vi "Set H Mode Torque.vi"(8 "error in (no error)":errorcluster, 10 "Torque_Reference_H":dbl, 11 "TCP modebus instance in":refnum<class "Modbus Master.lvclass">[](array[class])) -> (0 "error out":errorcluster, 3 "TCP modebus instance out":refnum<class "Modbus Master.lvclass">[](array[class]))   [LabVIEW 2025]
uses:
  <vilib>/Modbus/master/Modbus Master.lvclass
  C:/Program Files/National Instruments/LabVIEW 2025/vi.lib/Modbus/subvis/Modbus API/Modbus API.lvclass
  <vilib>/Modbus/subvis/Modbus API/Modbus API.lvclass/Modbus API.ctl
  <vilib>/Modbus/subvis/Transmission Data Unit (ADU)/Transmission Data Unit/Transmission Data Unit.lvclass/Transmission Data Unit.ctl
  <vilib>/Modbus/master/Data Access/Unit ID/Set Unit ID Property.vi
  <vilib>/Modbus/subvis/Transmission Data Unit (ADU)/Transmission Data Unit/Data Access/Unit ID/Write Unit ID.vi
  <vilib>/Modbus/subvis/Modbus API/Read Transmission Data Unit.vi
  <vilib>/Modbus/subvis/Modbus API/Write Transmission Data Unit.vi
  <vilib>/Modbus/subvis/Transmission Data Unit (ADU)/Transmission Data Unit/Transmission Data Unit.lvclass
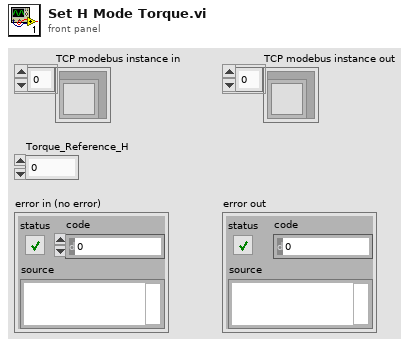
[diagram p1: front panel]
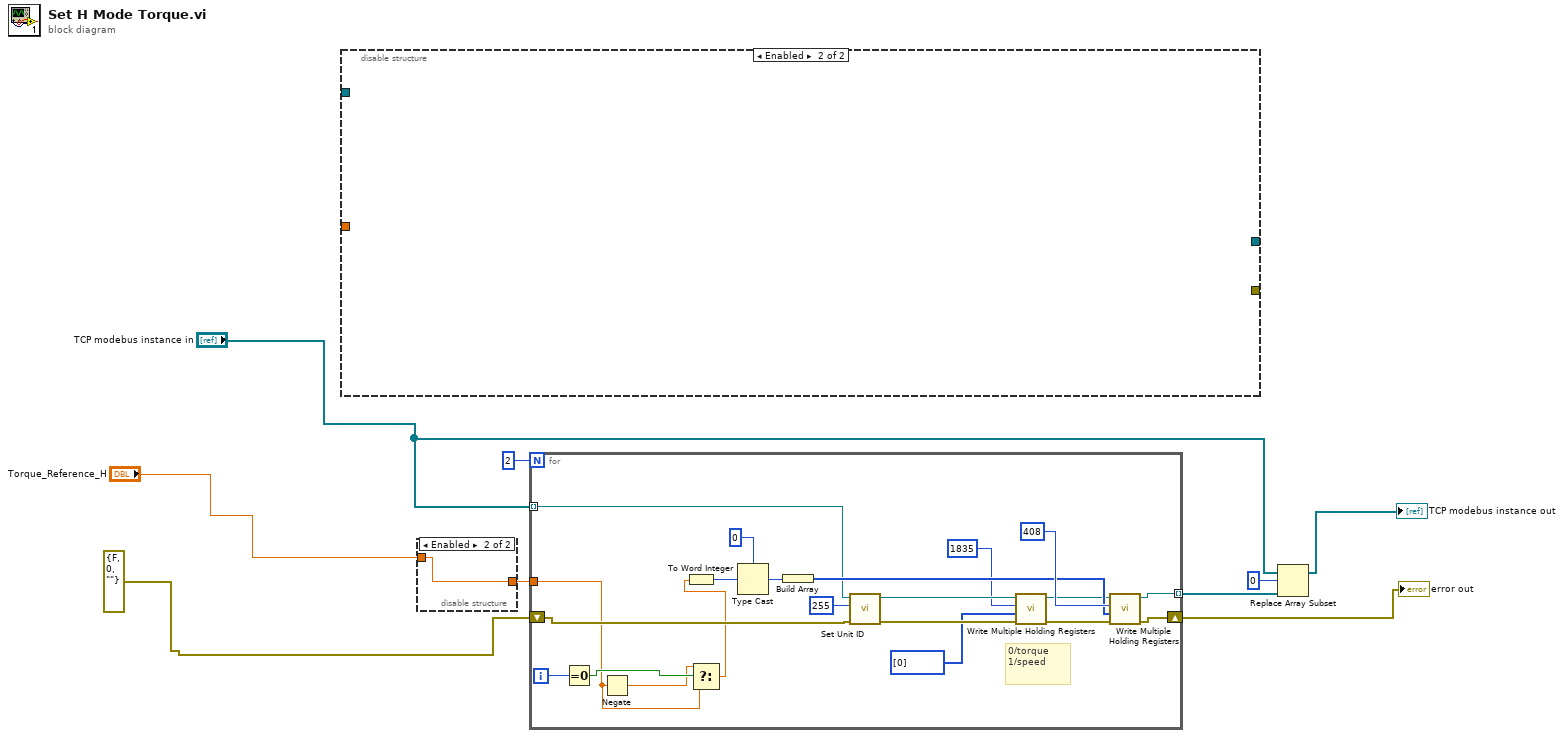
[diagram p0: block diagram]
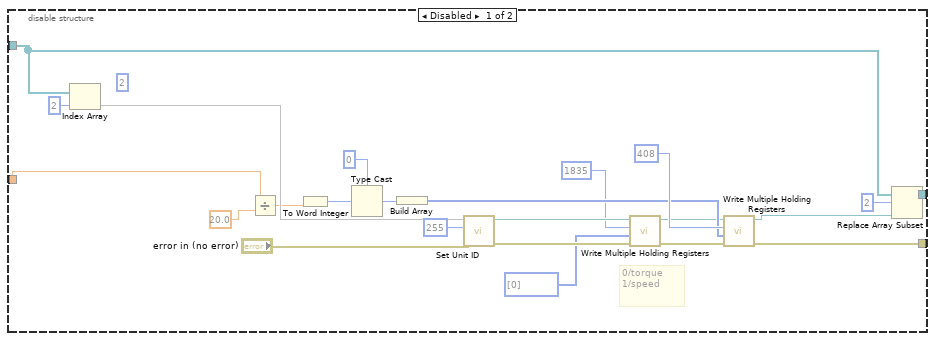
[diagram p2: hidden frame]
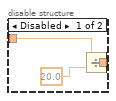
[diagram p3: hidden frame]
diagram:
  n1 = disable-structure shown="Enabled" {
    disable-tunnel: [w32 _] -> _
    disable-tunnel: _ -> [w29 _]
    disable-tunnel: [w28 _] -> _
    disable-tunnel: _ -> [w11 _]
    frame Disabled {
      (unwired) 2
      # "0/torque\n1/speed"
      n2 = Index Array(array=w11, index=2) -> (element=w12)
      n3 = Divide(x=w29, y=20.0) -> (x/y=w10:dbl)
      n4 = To Word Integer(number=w10) -> (16bit integer=w23:i16)
      n5 = Type Cast(type=u16 0, x=w23) -> (*(type *) &x=w24:u16)
      n6 = Build Array(w24) -> (w20:u16[])
      n7 = call <vilib>:"Set Unit ID.vi"("error in (no error)"="error in (no error)", "unit ID"=u8 255, "Modbus master in"=w12) -> ("error out"=w19:errorcluster, "Modbus master out"=w17:refnum<class "Modbus Master.lvclass">)  [unwired: 7 in]
      n8 = call-dynamic "Write Multiple Holding Registers.vi"("error in (no error)"=w19, "holding register values"=u16[] [0], "starting address"=u16 1835, "Modbus master in"=w17) -> ("error out"=w18:errorcluster, "Modbus master out"=w16:refnum<class "Modbus Master.lvclass">)  [unwired: 6 in]
      n9 = call-dynamic "Write Multiple Holding Registers.vi"("error in (no error)"=w18, "holding register values"=w20, "starting address"=u16 408, "Modbus master in"=w16) -> ("error out"=w28:errorcluster, "Modbus master out"=w30:refnum<class "Modbus Master.lvclass">)  [unwired: 6 in]
      n10 = Replace Array Subset(array=w11, new element=w30, index=2) -> (w32:refnum<class "Modbus Master.lvclass">[])
    }
    frame Enabled {
    }
  }
  n11 = disable-structure shown="Enabled" {
    disable-tunnel: [w35 w36] -> w9
    disable-tunnel: "Torque_Reference_H" -> [w34 w36]
    frame Disabled {
      n12 = Divide(x=w34, y=20.0) -> (x/y=w35:dbl)
    }
    frame Enabled {
    }
  }
  n13 = for {
    N: 2 -> [_]
    tunnel: w9 -> [w37]
    shift-right: [w50] -> w2
    shift-left: errorcluster {"status"=FALSE, "code"=0, "source"=""} ("error in (no error)") -> [w51]
    tunnel: "TCP modebus instance in" -> [w49] mode=indexing
    tunnel: [w48] -> w7 mode=indexing
    i -> [w47]
    # "0/torque\n1/speed"
    n14 = Equal To 0?(x=w47) -> (x = 0?=w39:bool)
    n15 = Negate(x=w37) -> (-x=w38:dbl)
    n16 = Select(t=w38, s=w39, f=w37) -> (s? t:f=w46:dbl)
    n17 = To Word Integer(number=w46) -> (16bit integer=w55:i16)
    n18 = Type Cast(type=u16 0, x=w55) -> (*(type *) &x=w56:u16)
    n19 = Build Array(w56) -> (w52:u16[])
    n20 = call <vilib>:"Set Unit ID.vi"("error in (no error)"=w51, "unit ID"=u8 255, "Modbus master in"=w49) -> ("error out"=w45:errorcluster, "Modbus master out"=w43:refnum<class "Modbus Master.lvclass">)  [unwired: 7 in]
    n21 = call-dynamic "Write Multiple Holding Registers.vi"("error in (no error)"=w45, "holding register values"=u16[] [0], "starting address"=u16 1835, "Modbus master in"=w43) -> ("error out"=w44:errorcluster, "Modbus master out"=w42:refnum<class "Modbus Master.lvclass">)  [unwired: 6 in]
    n22 = call-dynamic "Write Multiple Holding Registers.vi"("error in (no error)"=w44, "holding register values"=w52, "starting address"=u16 408, "Modbus master in"=w42) -> ("error out"=w50:errorcluster, "Modbus master out"=w48:refnum<class "Modbus Master.lvclass">)  [unwired: 6 in]
  }
  "error out" <- w2
  n23 = Replace Array Subset(array="TCP modebus instance in", new element=w7, index=0) -> (→"TCP modebus instance out":refnum<class "Modbus Master.lvclass">[])
